vi "Read Compatible Hardware Types.vi"(8 "error in (no error)":errorcluster, 11 "Voltage in":refnum<class "Frequency Measurement.lvclass">) -> (0 "error out":errorcluster, 2 "Compatible Hardware Types":string[](array[string]), 3 "Voltage out":refnum<class "Frequency Measurement.lvclass">)   [LabVIEW 2013, in "Frequency Measurement.lvlib" / "Frequency Measurement.lvclass"]
uses:
  Frequency Measurement.lvclass
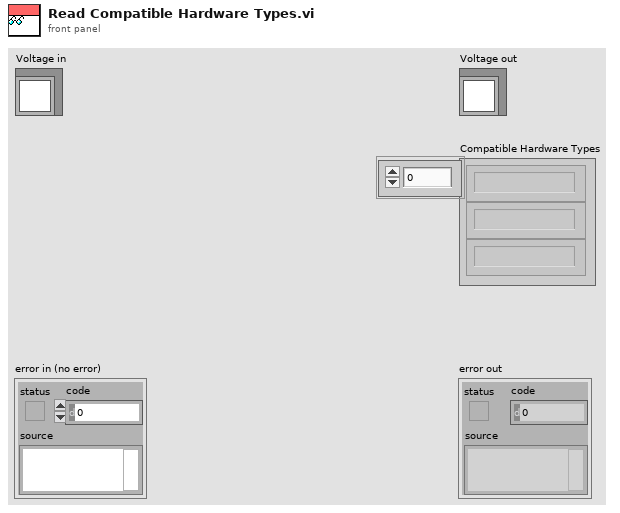
[diagram p1: front panel]
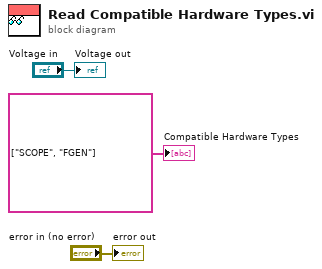
[diagram p0: block diagram]
diagram:
  "error out" <- "error in (no error)"
  "Voltage out" <- "Voltage in"
  "Compatible Hardware Types" <- string[] ["SCOPE", "FGEN"] ("Compatible Hardware Types")
